vi "Get Baseline Page Info.vi"(8 "error in 2":errorcluster, 9 "Tiff Bitness":T4(ring), 10 "Page Info":T3 {"Tags"."DataOffset" format="%x"}, 11 "Byte Stream File in":refnum<file>) -> (0 "error out":errorcluster, 1 "IFDO Info":T2(c390), 2 "Page Info":T5 {"SampleFormat" items=["UINT"=1, "INT"=2, "FP"=3, "VOID"=4, "COMPLEXINT"=5, "COMPLEXFP"=6]; "NewSubFileType" items=["FILETYPE_REDUCEDIMAGE"=1, "FILETYPE_PAGE"=2, "FILETYPE_MASK"=4]; "Compression" items=["COMPRESSION_NONE"=1, "COMPRESSION_CCITTRLE"=2, "COMPRESSION_CCITTFAX3"=3, "COMPRESSION_CCITTFAX4"=4, "COMPRESSION_LZW"=5, "COMPRESSION_OJPEG"=6, "COMPRESSION_JPEG"=7, "COMPRESSION_NEXT"=32766, "COMPRESSION_CCITTRLEW"=32771, "COMPRESSION_PACKBITS"=32773, "COMPRESSION_THUNDERSCAN"=32809, "COMPRESSION_IT8CTPAD"=32895, "COMPRESSION_IT8LW"=32896, "COMPRESSION_IT8MP"=32897, "COMPRESSION_IT8BL"=32898, "COMPRESSION_PIXARFILM"=32908, "COMPRESSION_PIXARLOG"=32909, "COMPRESSION_DEFLATE"=32946, "COMPRESSION_ADOBE_DEFLATE"=8, "COMPRESSION_DSC"=32947, "COMPRESSION_JBIG"=34661, "COMPRESSION_SGILOG"=34676, "COMPRESSION_SGILOG24"=34677, "COMPRESSION_JP2000"=34712]; "PhotometricInterpretation" items=["PHOTOMETRIC_MINISWHITE"=0, "PHOTOMETRIC_MINISBLACK"=1, "PHOTOMETRIC_RGB"=2, "PHOTOMETRIC_PALETTE"=3, "PHOTOMETRIC_MASK"=4, "PHOTOMETRIC_SEPARATED"=5, "PHOTOMETRIC_YCBCR"=6, "PHOTOMETRIC_CIELAB"=8, "PHOTOMETRIC_ICCLAB"=9, "PHOTOMETRIC_ITULAB"=10, "PHOTOMETRIC_LOGL"=32844, "PHOTOMETRIC_LOGLUV"=32845, "CFA"=32803, "LinearRaw"=34892, "DEPTH"=51177]; "ResolutionUnit" items=["RESUNIT_NONE"=1, "RESUNIT_INCH"=2, "RESUNIT_CENTIMETER"=3]}, 3 "Byte Stream File out":refnum<file>)   [LabVIEW 2020, in "LV Tiff.lvlib"]
uses:
  LV Tiff.lvlib
  Baseline Tags 1.ctl
  Tiff Data Type.ctl
  Tiff Tags.ctl
  <vilib>/Utility/Data Type/Type Definitions/Data Type.ctl
  <vilib>/Utility/Data Type/NI_Data Type.lvlib
panel:
  out "Variant":variant
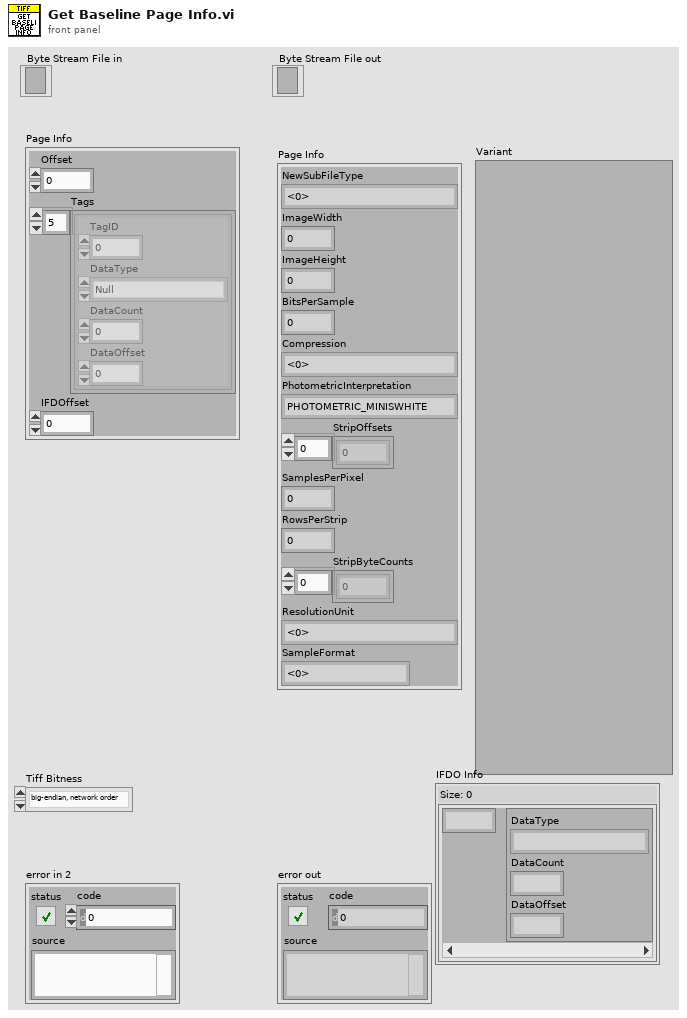
[diagram p1: front panel]
types:
  T1 = typedef "LV Tiff.lvlib/Tiff Data Type.ctl" = enum16{"Null", "BYTE", "ASCII", "SHORT", "LONG", "RATIONAL", "SBYTE", "UNDEFINE", "SSHORT", "SLONG", "SRATIONAL", "FLOAT", "DOUBLE"}
  T2 = map{u16, cluster{"DataType":T1, "DataCount":u32, "DataOffset":u32}}
  T3 = cluster{"Offset":i32, "Tags":cluster{"TagID":u16, "DataType":T1, "DataCount":u32, "DataOffset":u32}[], "IFDOffset":u32}
  T4 = enum16{"big-endian, network order", "native, host order", "little-endian"}
  T5 = typedef "LV Tiff.lvlib/Baseline Tags 1.ctl" = cluster{"NewSubFileType":u32, "ImageWidth":u32, "ImageHeight":u32, "BitsPerSample":u16, "Compression":u16, "PhotometricInterpretation":u16, "StripOffsets":u32[], "SamplesPerPixel":u16, "RowsPerStrip":u32, "StripByteCounts":u32[], "ResolutionUnit":u16, "SampleFormat":u16}
  T6 = typedef "LV Tiff.lvlib/Tiff Tags.ctl" = u16
  T7 = cluster{"TagID":u16, "DataType":T1, "DataCount":u32, "DataOffset":u32}[]
  T8 = cluster{"DataType":T1, "DataCount":u32, "DataOffset":u32}
  T9 = typedef "NI_Data Type.lvlib/Data Type.ctl" = enum8{"Invalid Type", "Void", "I8", "I16", "I32", "I64", "U8", "U16", "U32", "U64", "Single Float", "Double Float", "Extended Float", "Single Complex", "Double Complex", "Extended Complex", "Enum U8", "Enum U16", "Enum U32", "Enum U64", "Single Float With Unit", "Double Float With Unit", "Extended Float With Unit", "Single Complex with Unit", "Double Complex with Unit", "Extended Complex with Unit", "Boolean", "String", "Path", "Picture", "Tag", "Array", "Cluster", "Variant", "LV Variant", "Waveform", "Timestamp", "Digital Waveform", "Digital Data", "ExpressData", "Refnum", "External Data", "VI", "Poly VI", "LabVIEW Class Instance", "Fixed Point", "Set Collection", "Map Collection"}
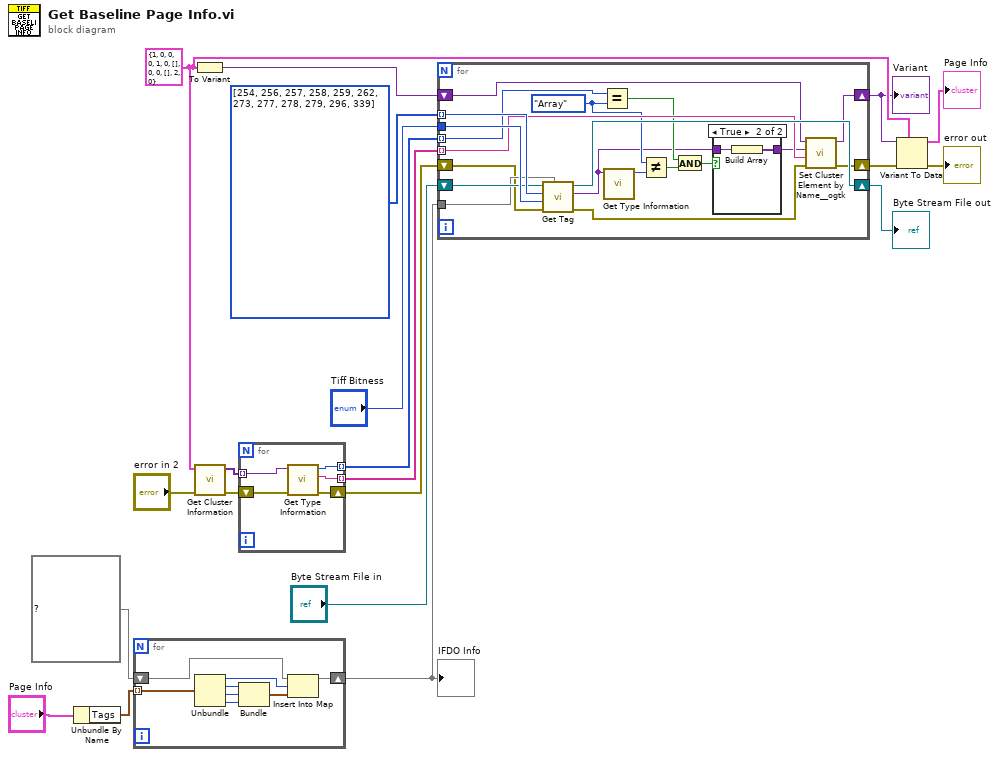
[diagram p0: block diagram]
diagram:
  w19 = T5 {"NewSubFileType"=1, "ImageWidth"=0, "ImageHeight"=0, "BitsPerSample"=0, "Compression"=1, "PhotometricInterpretation"=0, "StripOffsets"=[], "SamplesPerPixel"=0, "RowsPerStrip"=0, "StripByteCounts"=[], "ResolutionUnit"=2, "SampleFormat"=0}
  w11 = T6[] [254, 256, 257, 258, 259, 262, 273, 277, 278, 279, 296, 339] items=["NewSubfileType"=254, "ImageWidth"=256, "ImageLength"=257, "BitsPerSample"=258, "Compression"=259, "PhotometricInterpretation"=262, "StripOffsets"=273, "SamplesPerPixel"=277, "RowsPerStrip"=278, "StripByteCounts"=279, "XResolution"=282, "YResolution"=283, "ResolutionUnit"=296, "ColorMap"=320, "PlanarrConfiguration"=284, "YCbCrCoefficients"=529, "YCbCrSubSampling"=530, "YCbCrPositioning"=531, "ReferenceBlackWhite"=532, "BadFaxLines"=326, "CleanFaxData"=327, "ConsecutiveBadFaxLines"=328, "SampleFormat"=339]
  n1 = Unbundle By Name("Page Info") -> ("Tags"=w5:T7)
  n2 = for {
    tunnel: w5 -> [w28] mode=indexing
    shift-right: [w23] -> w14
    shift-left: T2 {} ("Map") -> [w24]
    n3 = Unbundle(w28) -> ("TagID"=w21:u16, "DataType"=w27:T1, "DataCount"=w26:u32, "DataOffset"=w25:u32)
    n4 = Bundle("DataType"=w27, "DataCount"=w26, "DataOffset"=w25) -> (w22:T8)  [unwired: 1 in]
    n5 = Insert Into Map(map in=w24, key=w21, value=w22) -> (map out=w23:T2)  [unwired: 2 out]
  }
  "IFDO Info" <- w14
  n6 = To Variant(anything=w19) -> (Variant=w17:variant)
  n7 = call <vilib>:"Get Cluster Information.vi"("error in (no error)"="error in 2", "variant"=w19) -> ("error out"=w2:errorcluster, "cluster elements"=w15:variant[])  [unwired: 8 in]
  n8 = for {
    tunnel: w15 -> [w33] mode=indexing
    tunnel: [w32] -> w16 mode=indexing
    tunnel: [w31] -> w4 mode=indexing
    shift-right: [w29] -> w1
    shift-left: w2 -> [w30]
    n9 = call <vilib>:"Get Type Information.vi"("error in (no error)"=w30, "variant"=w33) -> ("error out"=w29:errorcluster, "name"=w32:string, "type"=w31:T9)  [unwired: 5 in, 2 out]
  }
  n10 = for {
    tunnel: w11 -> [w52] mode=indexing
    tunnel: "Tiff Bitness" -> [w51]
    shift-right: [w50] -> w9
    shift-left: "Byte Stream File in" -> [w49]
    tunnel: w14 -> [w48]
    tunnel: w16 -> [w46] mode=indexing
    shift-right: [w47] -> w18
    shift-left: w17 -> [w37]
    shift-right: [w43] -> w8
    shift-left: w1 -> [w45]
    tunnel: w4 -> [w34] mode=indexing
    w42 = Data_Type."Array" ("y")
    n11 = call "Get Tag.vi"("IFDO"=w48, "error in 2"=w45, "byte order (0:big-endian, network order)"=w51, "Tag ID"=w52, "File Refnum"=w49) -> ("error out"=w44:errorcluster, "Data"=w36:variant, "refnum out"=w50:refnum<file>)  [unwired: 3 in, 1 out]
    n12 = Equal?(x=w34, y=w42) -> (x = y?=w40:bool)
    n13 = call <vilib>:"Get Type Information.vi"("variant"=w36) -> ("type"=w41:T9)  [unwired: 6 in, 4 out]
    n14 = Not Equal?(x=w42, y=w41) -> (x != y?=w39:bool)
    n15 = And(x=w40, y=w39) -> (x .and. y?=w38:bool)
    n16 = case shown="True" w38 {
      tunnel: [w53 w54] -> w35
      tunnel: w36 -> [w53 w55]
      frame False {
      }
      frame True {
        n17 = Build Array(w55) -> (w54:variant[])
      }
    }
    n18 = call <userlib>:"Set Cluster Element by Name__ogtk.vi"("error in (no error)"=w44, "Element Name (\"\": New Element Data Name)"=w46, "New Element Value"=w35, "Cluster"=w37) -> ("error out"=w43:errorcluster, "VCluster out"=w47:variant)  [unwired: 5 in, 1 out]
  }
  "Byte Stream File out" <- w9
  "Variant" <- w18
  n19 = Variant To Data(error in=w8, type=w19, Variant=w18) -> (data=→"Page Info":T5, error out=→"error out":errorcluster)
